vi "Configure Output Protection WDog Delay.vi"(8 "error in (no error)":errorcluster, 10 "Time(0)":dbl, 11 "VISA resource name":refnum<visa-resource-name>) -> (0 "error out":errorcluster, 3 "VISA resource name out":refnum<visa-resource-name>)   [LabVIEW 2020, in "IT6000C.lvlib"]
doc: "This command is used to set the software watchdog timeout, or monitor latency.When monitor timer is enabled, output is disabled if there is no SCPI I/O activity on all remote interfaces during the latency.The monitor timer function is not reset by the activity on the front panel, and the output continues to shut down after this interval has passed.Values range programmatically from 1 to 3600 seconds, incrementing each time by 1 second."
uses:
  IT6000C.lvlib
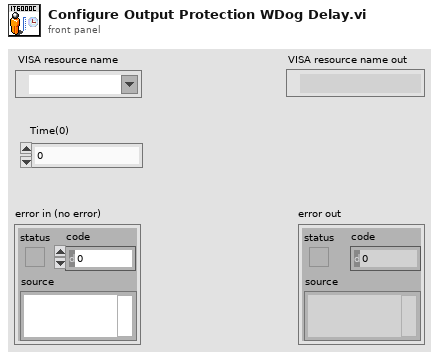
[diagram p1: front panel]
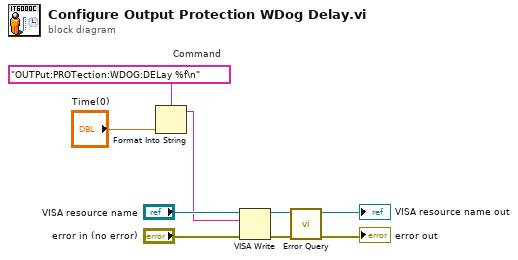
[diagram p0: block diagram]
diagram:
  w3 = "OUTPut:PROTection:WDOG:DELay %f\n"  # Command
  n1 = Format Into String(format string=w3, "Time(0)") -> (resulting string=w1:string)  [unwired: 2 in, 1 out]
  n2 = VISA Write(VISA resource name="VISA resource name", write buffer=w1, error in (no error)="error in (no error)") -> (VISA resource name out=w6:refnum<visa-resource-name>, error out=w7:errorcluster)  [unwired: 1 out]
  n3 = call "Error Query.vi"("error in (no error)"=w7, "VISA resource name"=w6) -> ("error out"=→"error out":errorcluster, "VISA resource name out"=→"VISA resource name out":refnum<visa-resource-name>)  [unwired: 6 in, 2 out]
